vi "Dashboard Main.vi"() -> ()   [LabVIEW 2018]
uses:
  <vilib>/Rock Robotics/WPI/Camera/WPI_CameraSettings Read MJPG.ctl
  <vilib>/Rock Robotics/WPI/Camera/WPI_CameraImageSize.ctl
  <vilib>/Rock Robotics/WPI/Camera/WPI_CameraExposure Values.ctl
  <vilib>/Rock Robotics/WPI/Camera/WPI_CameraWhite Balance Values.ctl
  <vilib>/Utility/miscctls.llb/LVRowAndColumnTypeDef.ctl
  <vilib>/event_ctls.llb/eventvkey.ctl
  <vilib>/Rock Robotics/Network Tables/NT Read Numeric Array.vi
  <vilib>/Rock Robotics/WPI/Dashboard/WPI_DashboardLogging Global.vi
  <vilib>/Rock Robotics/Network Tables/NT Write Boolean.vi
  Vision Things/Dashboard globals.vi
  <vilib>/Utility/inputDevices.llb/keyboardAcquire.vi
  <vilib>/Rock Robotics/Network Tables/NT Write Variant.vi
panel:
  out "Time Remaining":sgl
  in  "Camera Settings Right":T1={"Frame Rate"=30, "Compression"=30, "Size"=1, "DB Camera Config"=FALSE} {"Frame Rate" scale=1.0..30.0; "Compression" scale=100.0..-1.0; "Size" items=["640x480", "320x240", "160x120"]}
  in  "Camera Name Right":string(combo)="No Camera Selection"
  out "Camera Perf":string
  in  "Camera Settings":T1={"Frame Rate"=30, "Compression"=30, "Size"=1, "DB Camera Config"=FALSE} {"Frame Rate" scale=1.0..30.0; "Compression" scale=100.0..-1.0; "Size" items=["640x480", "320x240", "160x120"]}
  in  "TCP":refnum<k5>
  in  "Rec Mode":enum32{"Stop", "Record", "Playback"}(radio)
  out "Robot IP":string
  out "Image Message":string="Timeout in Camera Communications"
  in  "Dashboard Tab":T2(tab)
  in  "Don't do Auton":bool
  in  "Desired Target":T3(radio)
  in  "Select Auto":string(combo)="Select Autonomous ..."
  out "NT Connection":bool
  out "MotorChart R":cluster{"Numeric":dbl, "Numeric":dbl}(graph)
  out "MotorChart L":cluster{"Numeric":dbl, "Numeric":dbl}(graph)
  out "MotorSliders R":cluster{"MotorSlide1":dbl, "MotorSlide2":dbl} {"MotorSlide2" scale=-1.0..1.0 scale format="%#_2e"; "MotorSlide1" scale=-1.0..1.0 scale format="%#_2e"}
  out "MotorSliders L":cluster{"MotorSlide1":dbl, "MotorSlide2":dbl} {"MotorSlide2" scale=-1.0..1.0 scale format="%#_2e"; "MotorSlide1" scale=-1.0..1.0 scale format="%#_2e"}
  out "Gyro":dbl(knob) scale=0.0..360.0
  out "JS1 Z":dbl(slide) scale=-1.0..1.0 scale format="%#_2e"
  out "JS1 Graph":cluster{"X":dbl, "Y":dbl}[](graph)
  out "JS1 Buttons":T4
  out "JS2 Z":dbl(slide) scale=-1.0..1.0 scale format="%#_2e"
  out "JS2 Graph":cluster{"X":dbl, "Y":dbl}[](graph)
  out "JS2 Buttons":T4
  out "Mode":T5(ring)=enum."Auto Disabled"
  out "Right Camera Perf":cluster{"Bandwidth (Mbps)":dbl, "FPS":dbl}
  in  "Auton Side":enum16{"Front", "Left", "Right"}(ring)
  in  "Side Code":enum16{"Right", "Left"}(ring)
  in  "Slot #":enum16{"3", "2", "1"}(ring)
  out "Auton String":string
  in  "Starting Postion":enum16{"2R", "2L", "1L", "1R", "1M"}(ring)
  in  "Camera 0 Settings":T6={"fps"=30, "compression"=30, "Image Size"=enum."320x240", "Config Shown"=FALSE}
  in  "Camera 1 Settings":T6={"fps"=30, "compression"=30, "Image Size"=enum."320x240", "Config Shown"=FALSE}
  out "Camera Image Right":T8(plugin-control)
  in  "DB/String 9":string
  in  "DB/String 8":string
  in  "DB/String 7":string
  in  "DB/String 6":string
  in  "DB/String 5":string
  in  "DB/String 4":string
  in  "DB/String 3":string
  in  "DB/String 2":string
  in  "DB/String 1":string
  in  "DB/String 0":string
  in  "DB/Slider 0":dbl(slide) scale=0.0..5.0
  in  "DB/Slider 1":dbl(slide) scale=0.0..5.0
  in  "DB/Slider 2":dbl(slide) scale=0.0..5.0
  in  "DB/Slider 3":dbl(slide) scale=0.0..5.0
  out "DB/LED 3":bool
  out "DB/LED 2":bool
  out "DB/LED 1":bool
  out "DB/LED 0":bool
  in  "DB/Button 3":bool
  in  "DB/Button 2":bool
  in  "DB/Button 1":bool
  in  "DB/Button 0":bool caption="New Name"
  in  "Test Slider":dbl(slide) scale=0.0..100.0 scale format="%#_3g"
  in  "On/Off":bool caption="Solenoid"
  in  "Test Name":u16(ring) items=["Select the test to run..."]
  in  "Test Tree":string(tree)
  in  "Motor":cluster{"Value":dbl, "Enable":bool} {"Value" scale=-1.0..1.0 scale format="%#_3g"}
  out "Progress":T9 {"Test Progress" scale=0.0..100.0}
  in  "Rev/Fwd":cluster{"Forward":bool, "Reverse":bool}
  in  "Test Ring":u16(ring) items=["Monochrome", "Color"]
  out "Cmd Status":string
  in  "Execute Command":bool
  in  "Command Params":string[][](table)
  in  "Command Selection":i32(listbox)
  in  "CheckList":i32(listbox)
  out "Tree":string(tree)
  out "Camera Image":T8(plugin-control)
  out "Background":bool
  in  "Camera Name":string(combo)="No Camera Selection"
  # "HW"
  # "HW"
  # "Joysticks"
  # "Drive Motors"
  # "Front"
  # "Right"
  # "Left"
  # "Back"
  # "This Tab intentionally left empty"
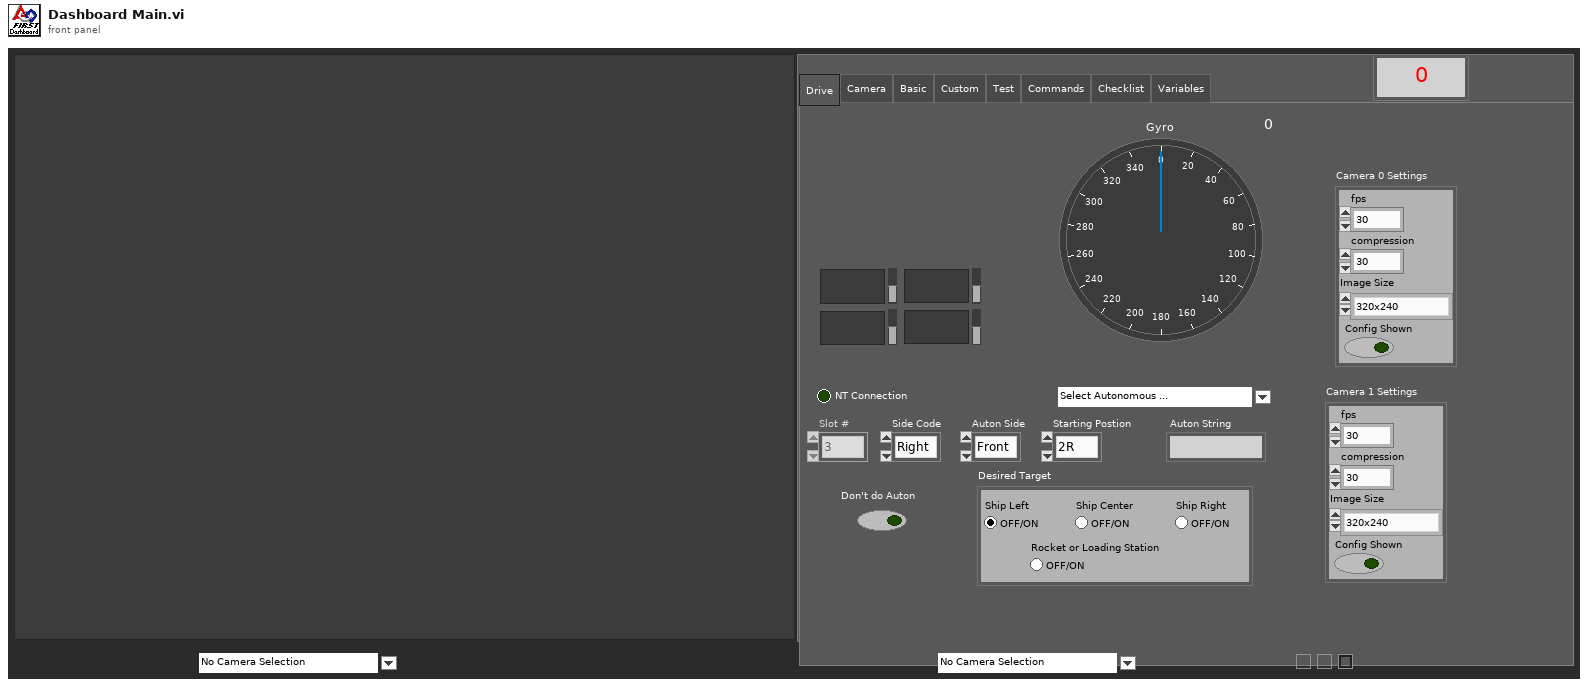
[diagram p1: front panel]
types:
  T1 = cluster{"Frame Rate":i32, "Compression":i32, "Size":u16, "DB Camera Config":bool}
  T2 = enum32{"Drive", "Camera", "Basic", "Custom", "Test", "Commands", "Checklist", "Variables"}
  T3 = enum32{"Ship Left", "Ship Center", "Ship Right", "Rocket or Loading Station"}
  T4 = cluster{bool, bool, bool, bool, bool, bool, bool, bool, bool, bool, bool, bool}
  T5 = enum8{"Tele-Op Disabled", "Tele-Op Enabled", "Auto Disabled", "Auto Enabled", "Test Disabled", "Test Enabled", "Disconnected", "No Code", "E-Stop"}
  T6 = typedef "WPI_CameraSettings Read MJPG.ctl" = cluster{"fps":i32, "compression":i32, "Image Size":T7, "Config Shown":bool}
  T7 = typedef "WPI_CameraImageSize.ctl" = enum16{"640x480", "320x240", "160x120", "Custom"}
  T8 = typedef "IMAQ Image.ctl" = refnum<image>
  T9 = cluster{"Test Progress":u8, "Test Progress Text":string}
  T10 = cluster{"Save Path":path, "Interval (s)":dbl, "Keep":i32}
  T11 = typedef "Image Type" = u32
  T12 = cluster{"IDs":cluster{"RPC field ID":u16, "Unique ID":u16}, "String":string}
  T13 = enum8{"Enabled", "Disabled", "Disabled and Grayed Out"}
  T14 = enum16{"0", "1", "2", "3", "4", "5", "6", "7", "8", "9", "A", "B", "C", "D", "E", "F", "G", "H", "I", "J", "K", "L", "M", "N", "O", "P", "Q", "R", "S", "T", "U", "V", "W", "X", "Y", "Z", "F1", "F2", "F3", "F4", "F5", "F6", "F7", "F8", "F9", "F10", "F11", "F12", "F13", "F14", "F15", "ADD", "BACK", "BACKSLASH", "CAPITAL", "COMMA", "DECIMAL", "DELETE", "DIVIDE", "DOWN", "END", "EQUALS", "ESCAPE", "GRAVE (`)", "HOME", "INSERT", "LBRACKET", "LCONTROL", "LEFT", "L ALT", "LSHIFT", "LWIN", "MINUS", "MULTIPLY", "NEXT", "NUMLOCK", "NUMPAD_0", "NUMPAD_1", "NUMPAD_2", "NUMPAD_3", "NUMPAD_4", "NUMPAD_5", "NUMPAD_6", "NUMPAD_7", "NUMPAD_8", "NUMPAD_9", "PAUSE", "PERIOD", "PRIOR (PG UP)", "RBRACKET", "RCONTROL", "RETURN", "RIGHT", "R ALT", "RSHIFT", "RWIN", "SCROLL", "SEMICOLON", "SLASH", "SPACE", "SUBTRACT", "TAB", "UP", "ENTER (num pad)", "' (quote)"}[]
  T15 = enum16{"0", "1", "2", "3", "4", "5", "6", "7", "8", "9", "A", "B", "C", "D", "E", "F", "G", "H", "I", "J", "K", "L", "M", "N", "O", "P", "Q", "R", "S", "T", "U", "V", "W", "X", "Y", "Z", "F1", "F2", "F3", "F4", "F5", "F6", "F7", "F8", "F9", "F10", "F11", "F12", "F13", "F14", "F15", "ADD", "BACK", "BACKSLASH", "CAPITAL", "COMMA", "DECIMAL", "DELETE", "DIVIDE", "DOWN", "END", "EQUALS", "ESCAPE", "GRAVE (`)", "HOME", "INSERT", "LBRACKET", "LCONTROL", "LEFT", "L ALT", "LSHIFT", "LWIN", "MINUS", "MULTIPLY", "NEXT", "NUMLOCK", "NUMPAD_0", "NUMPAD_1", "NUMPAD_2", "NUMPAD_3", "NUMPAD_4", "NUMPAD_5", "NUMPAD_6", "NUMPAD_7", "NUMPAD_8", "NUMPAD_9", "PAUSE", "PERIOD", "PRIOR (PG UP)", "RBRACKET", "RCONTROL", "RETURN", "RIGHT", "R ALT", "RSHIFT", "RWIN", "SCROLL", "SEMICOLON", "SLASH", "SPACE", "SUBTRACT", "TAB", "UP", "ENTER (num pad)", "' (quote)"}
  T16 = typedef "WPI_CameraExposure Values.ctl" = enum16{"Auto", "Flicker-free 50 Hz", "Flicker-free 60 Hz", "Hold current", "Custom"}
  T17 = typedef "WPI_CameraWhite Balance Values.ctl" = enum16{"Auto", "Fixed indoor", "Fixed outdoor 1", "Fixed outdoor 2", "Fixed fluorescent 1", "Fixed fluorescent 2", "Hold current", "Custom"}
  T18 = cluster{"Exposure":T16, "Exposure (%)":dbl, "Brightness":i32, "White Balance":T17, "Color Temp (K)":dbl}
  T19 = cluster{"Global Rectangle":i32[], "Contours":cluster{"Contour Type":u32, "ROI Type":u32, "Points":i32[]}[]}
  T20 = cluster{"Camera Name":string, string, "Saved DB Images Info":cluster{"Save Path":path, "Interval (s)":dbl, "Keep":i32}}
  T21 = cluster{"Camera Name Right":string, string, "Saved DB Images Info":cluster{"Save Path":path, "Interval (s)":dbl, "Keep":i32}}
  T22 = cluster{"Camera Image":refnum<vi>, "Dashboard Tab":refnum<vi>, "Background":refnum<vi>, "Rec Mode":refnum<vi>, "Test Slider":refnum<vi>, "On/Off ":refnum<vi>, "Test Ring":refnum<vi>, "Rev/Fwd":refnum<vi>, "Test Name":refnum<vi>, "Motor":refnum<vi>, "Progress":refnum<vi>, "CheckList":refnum<vi>, "Tree":refnum<vi>, "Test Tree":refnum<vi>, "Command Params":refnum<vi>, "Command Selection":refnum<vi>, "Execute Command":refnum<vi>, "Cmd Status":refnum<vi>, "Camera Settings":refnum<vi>, "Camera Name":refnum<vi>, "Camera Perf":refnum<vi>, "Camera Settings Right":refnum<vi>, "Camera Name Right":refnum<vi>, "Camera Image Right":refnum<vi>}
  T23 = cluster{"Error Strings":string, "Disable Counts":cluster{u16, u16}, "Rail Faults":cluster{u16, u16, u16}, "Robot IP":string, "DB Mode":u8, "Event Info":cluster{"Name":string, "Type":u8, "Number":u16, "Replay":u8}}
  T24 = cluster{"Storage":cluster{"Disk Free":u64, "RAM Block":u32, "RAM free":u32}, "CPU Utilization":cluster{"CPU % ISR":sgl, "CPU % Time Crit":sgl, "CPU % Timed Str":sgl, "CPU % High":sgl, "CPU % Above":sgl, "CPU % Normal":sgl, "CPU % Low":sgl}, "CAN":cluster{"% Bus Utilization":sgl, "Bus Off Cnt":u32, "TX_FIFO Full Cnt":u32, "Receive Error Cnt":u8, "Transmit Error Cnt":u8}, "HID":cluster{"HID Outputs":u32, "Rumble Low":u16, "Rumble High":u16}[]}
  T25 = cluster{"Status bits":cluster{"Test Mode":bool, "Autonomous":bool, "Enabled":bool, "Code Start":bool, "Brownout":bool, "Reserved 2":bool, "Reserved 3":bool, "E-Stop":bool}, "Code Trace":cluster{"Disabled":bool, "TeleOp":bool, "Auto":bool, "Test":bool}, "Controller Type":enum16{"unknown", "cRIO", "roboRio"}, "Code?":enum16{"unknown", "noCode", "code"}, "Battery V":dbl}
  T26 = cluster{"Control Bits":cluster{"TestMode":bool, "Autonomous":bool, "Enabled":bool, "FMS Present":bool, bool, bool, bool, "E-Stop":bool}, "Team Station ":u8, "Countdown":sgl, "Joystick Values":cluster{"Axes":dbl[], "Buttons":bool[], "POVs":i16[]}[]}
  T27 = cluster{"Increase in Left":dbl, "Increase in Right":dbl}[]
  T28 = cluster{"Axes":dbl[], "Buttons":bool[], "POVs":i16[]}[]
  T29 = cluster{"Axes":dbl[], "Buttons":bool[], "POVs":i16[]}
  T30 = cluster{"Buttons[0]":bool, "Buttons[1]":bool, "Buttons[2]":bool, "Buttons[3]":bool, "Buttons[4]":bool, "Buttons[5]":bool, "Buttons[6]":bool, "Buttons[7]":bool, "Buttons[8]":bool, "Buttons[9]":bool, "Buttons[10]":bool, "Buttons[11]":bool}
  T31 = cluster{"Operation":enum16{"Update", "Clear"}, "Color Box":u32}[]
  T32 = typedef "eventvkey.ctl" = enum16{"ASCII", "Enter", "Return", "Shift", "Ctrl", "Alt", "Cmd", "Opt", "Caps", "NumLock", "Clear", "Break", "Up", "Down", "Left", "Right", "Insert", "Delete", "Home", "End", "PageUp", "PageDown", "Escape", "Help", "Pause", "ScrollLock", "F1", "F2", "F3", "F4", "F5", "F6", "F7", "F8", "F9", "F10", "F11", "F12", "F13", "F14", "F15", "F16", "F17", "F18", "F19", "F20", "F21", "F22", "F23", "F24", "Play", "VolumeUp", "VolumeDown", "Mute", "Two Byte Char"}
  T33 = cluster{"Image Size":bool, "Image Type":bool, "Pixel Value":bool, "ROI Information":bool, "Zoom Factor":bool}
  T34 = cluster{"Operation":enum16{"Update", "Clear"}, "Color Box":u32}
  T35 = typedef "LVRowAndColumnTypeDef.ctl" = cluster{"Row":i32, "Column":i32}
  T36 = cluster{"Shift":bool, "Ctrl":bool, "Alt":bool, "Cmd":bool, "Opt":bool}
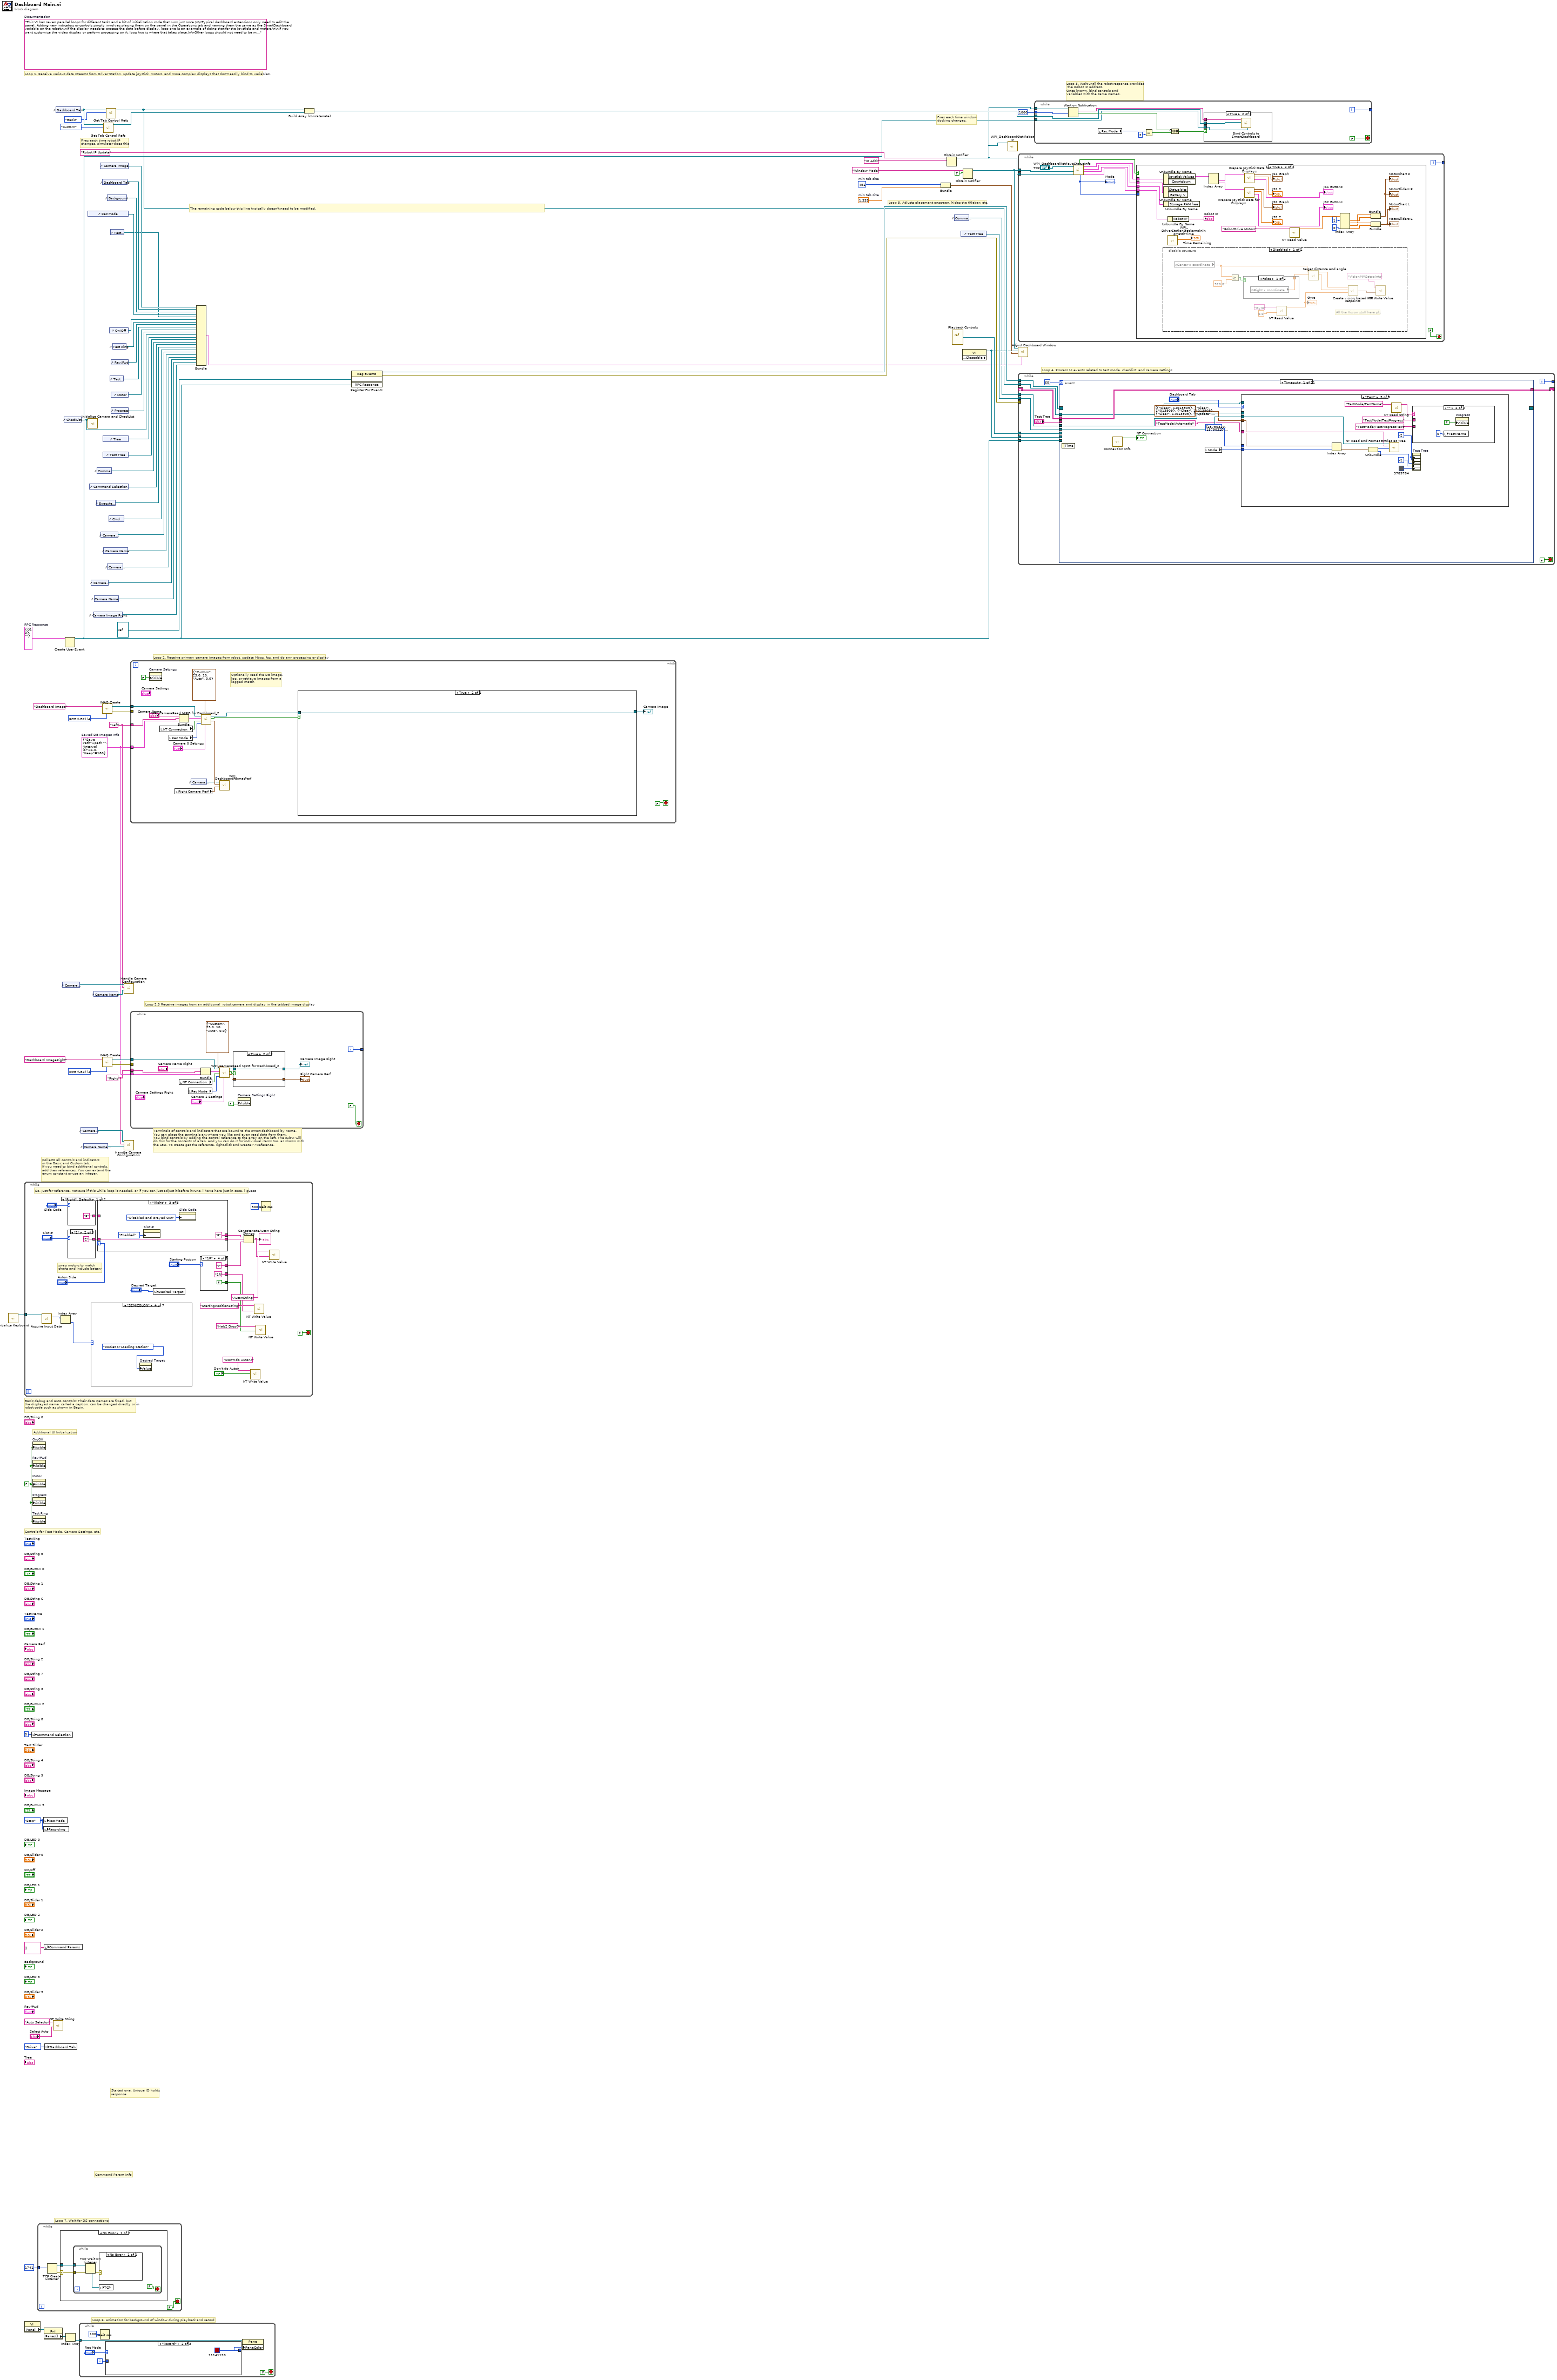
[diagram p0: block diagram]
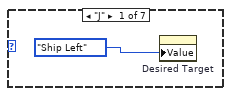
[diagram p2: hidden frame]
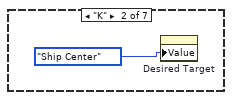
[diagram p3: hidden frame]
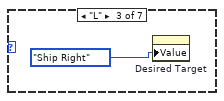
[diagram p4: hidden frame]
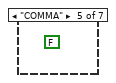
[diagram p5: hidden frame]
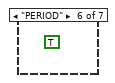
[diagram p6: hidden frame]
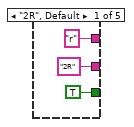
[diagram p8: hidden frame]
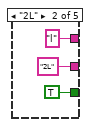
[diagram p9: hidden frame]
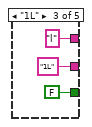
[diagram p10: hidden frame]
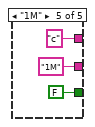
[diagram p11: hidden frame]
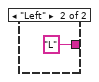
[diagram p12: hidden frame]
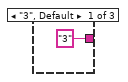
[diagram p13: hidden frame]
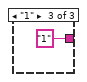
[diagram p14: hidden frame]
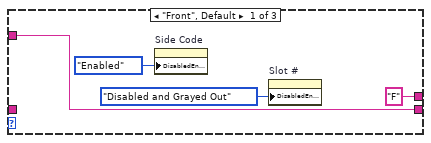
[diagram p15: hidden frame]
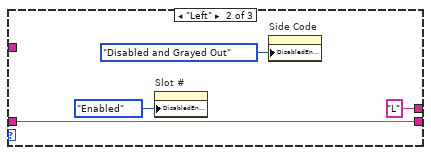
[diagram p16: hidden frame]
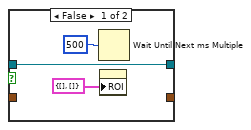
[diagram p17: hidden frame]
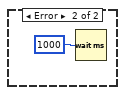
[diagram p18: hidden frame]
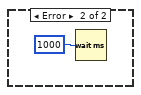
[diagram p19: hidden frame]
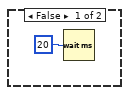
[diagram p20: hidden frame]
diagram:
  w5 = T10 {"Save Path"=path "", "Interval (s)"=1.0, "Keep"=180}  # Saved DB Images Info
  w4 = "Right"
  w3 = "Left"
  w15 = T11 4 items=["Grayscale (U8)", "Grayscale (I16)", "Grayscale (SGL)", "Complex (CSG)", "RGB (U32)", "HSL (U32)", "RGB (U64)"] ("Image Type")
  w31 = T12 {"IDs"={"RPC field ID"=0, "Unique ID"=0}, "String"=""}  # RPC Response
  w53 = 491  # min tab size
  w52 = 1.333  # min tab size
  w60 = enum32{"Stop", "Record", "Playback"}."Stop" ("Rec Mode")
  w37 = FALSE ("Visible")
  (unwired) "This VI has seven parallel loops for different tasks and a bit of initialization code that runs just once.\n\nTypical dashboard extensions only need to edit the panel. Adding new indicators or controls simply involves placing them on the panel in the Operations tab and naming them the same as the SmartDashboard variable on the robot\n\nIf the display needs to process the data before display, loop one is an example of doing that for the joysticks and motors.\n\nIf you want customize the video display or perform processing on it, loop two is where that takes place.\n\nOther loops should not need to be modified. They are pretty standard, and document the task they perform."  # Documentation
  w77 = T11 4 items=["Grayscale (U8)", "Grayscale (I16)", "Grayscale (SGL)", "Complex (CSG)", "RGB (U32)", "HSL (U32)", "RGB (U64)"] ("Image Type")
  # "Collects all controls and indicators\nin the Basic and Custom tab.\nIf you need to bind additional controls,\nadd their references. You can extend the\nenum constant or use an integer."
  # "Terminals of controls and indicators that are bound to the smart dashboard by name.\nYou can place the terminals anywhere you like and even read data from them.\nYou bind controls by adding the control reference to the array on the left. The subVI will\ndo this for the contents of a tab, and you can do it for individual items too, as shown with\nthe LED. To create get the reference, right-click and Create>>Reference."
  # "Loop 2.5 Receive images from an additional  robot camera and display in the tabbed image display"
  # "Command Param Info"
  # "Started one, Unique ID holds\nresponse"
  # "Loop 7. Wait for DS connections"
  # "Basic debug and auto controls: Their data names are fixed, but\nthe displayed name, called a caption, can be changed directly or in\nrobot code such as shown in Begin."
  # "Controls for Test Mode, Camera Settings, etc."
  # "Additional UI Initialization"
  # "Loop 6. Animation for background of window during playback and record"
  # "Fires each time robot IP\nchanges, simulator does this"
  # "Fires each time window\ndocking changes."
  # "The remaining code below this line typically doesn't need to be modified."
  # "Loop 4. Process UI events related to test mode, checklist, and camera settings"
  # "Loop 3. Wait until the robot response provides\n the Robot IP address.\nOnce known, bind controls and\nvariables with the same names."
  # "Loop 5. Adjusts placement onscreen, hides the titlebar, etc."
  # "Loop 1. Receive various data streams from Driver Station, update joystick, motors, and more complex displays that don't easily bind to variables."
  # "Loop 2. Receive primary camera images from robot, update Mbps, fps, and do any processing or display"
  n1 = call <vilib>:"Intialize Keyboard.vi"() -> ("device ID"=w2:refnum<k1>)  [unwired: 10 in, 1 out]
  n2 = while {
    tunnel: w2 -> [w84]
    stop <- FALSE stop-if-true
    # "So, Just for reference, not sure if this while loop is needed, or if you can just adjust it before it runs, i have here just in case, i guess"
    # "swap motors to match\ncharts and include battery"
    n3 = call-poly <vilib>:"Acquire Input Data.vi"("device ID"=w84) -> ("keys pressed"=w83:T14)  [unwired: 16 in, 2 out]
    n4 = Index Array(array=w83) -> (element=w82:T15)  [unwired: 1 in]
    n5 = case shown="\"Right\", Default" "Side Code" {
      tunnel: ["R" "L"] -> w96
      frame "Right", Default {
      }
      frame "Left" {
      }
    }
    n6 = case shown="\"2\"" "Slot #" {
      tunnel: ["3" "2" "1"] -> w97
      frame "3", Default {
      }
      frame "2" {
      }
      frame "1" {
      }
    }
    n7 = case shown="\"SEMICOLON\"" w82 {
      frame "J" {
        n8 = property on="Desired Target" class="RadioBtnsControl (strict)"("Value"=T3."Ship Left" ("Desired Target")) -> ()  [unwired: 2 in, 2 out]
      }
      frame "K" {
        n9 = property on="Desired Target" class="RadioBtnsControl (strict)"("Value"=T3."Ship Center" ("Desired Target")) -> ()  [unwired: 2 in, 2 out]
      }
      frame "L" {
        n10 = property on="Desired Target" class="RadioBtnsControl (strict)"("Value"=T3."Ship Right" ("Desired Target")) -> ()  [unwired: 2 in, 2 out]
      }
      frame "SEMICOLON" {
        n11 = property on="Desired Target" class="RadioBtnsControl (strict)"("Value"=T3."Rocket or Loading Station" ("Desired Target")) -> ()  [unwired: 2 in, 2 out]
      }
      frame "COMMA" {
        (unwired) FALSE ("Enable Vision Processing")
      }
      frame "PERIOD" {
        (unwired) TRUE ("Enable Vision Processing")
      }
      frame "0", Default {
      }
    }
    n12 = case shown="\"Right\"" "Auton Side" {
      tunnel: w97 -> [_ w129 w133]
      tunnel: w96 -> [w125 _ _]
      tunnel: [w125 w129 w133] -> w92
      tunnel: ["F" "L" "R"] -> w93
      frame "Front", Default {
        n13 = property on="Side Code" class="Enum (strict)"("DisabledEnum"=T13."Enabled" ("Disabled")) -> ()  [unwired: 2 in, 2 out]
        n14 = property on="Slot #" class="Enum (strict)"("DisabledEnum"=T13."Disabled and Grayed Out" ("Disabled")) -> ()  [unwired: 2 in, 2 out]
      }
      frame "Left" {
        n15 = property on="Slot #" class="Enum (strict)"("DisabledEnum"=T13."Enabled" ("Disabled")) -> ()  [unwired: 2 in, 2 out]
        n16 = property on="Side Code" class="Enum (strict)"("DisabledEnum"=T13."Disabled and Grayed Out" ("Disabled")) -> ()  [unwired: 2 in, 2 out]
      }
      frame "Right" {
        n17 = property on="Slot #" class="Enum (strict)"("DisabledEnum"=T13."Enabled" ("Disabled")) -> ()  [unwired: 2 in, 2 out]
        n18 = property on="Side Code" class="Enum (strict)"("DisabledEnum"=T13."Disabled and Grayed Out" ("Disabled")) -> ()  [unwired: 2 in, 2 out]
      }
    }
    n19 = global write "Dashboard globals.vi" "Desired Target"("Desired Target") -> ()
    n20 = case shown="\"1R\"" "Starting Postion" {
      tunnel: ["2R" "2L" "1L" "1R" "1M"] -> w89
      tunnel: [TRUE TRUE FALSE FALSE FALSE] -> w86
      tunnel: ["r" "l" "l" "r" "c"] -> w85
      frame "2R", Default {
      }
      frame "2L" {
      }
      frame "1L" {
      }
      frame "1R" {
      }
      frame "1M" {
      }
    }
    n21 = Concatenate Strings(w93, w92, w85) -> (w90:string)
    "Auton String" <- w90
    n22 = call-poly <vilib>:"NT Write Value.vi"("Boolean"="Don't do Auton", "Name"="Don't do Auton?") -> ()  [unwired: 9 in, 1 out]
    n23 = call-poly <vilib>:"NT Write Value.vi"("String"=w89, "Name"="StartingPositionString") -> ()  [unwired: 9 in, 1 out]
    n24 = call-poly <vilib>:"NT Write Value.vi"("Boolean"=w86, "Name"="Hab2 Drop?") -> ()  [unwired: 9 in, 1 out]
    n25 = Wait (ms)(milliseconds to wait=u32 500) -> ()  [unwired: 1 out]
    n26 = call-poly <vilib>:"NT Write Value.vi"("String"=w90, "Name"="AutonString") -> ()  [unwired: 9 in, 1 out]
  }
  n27 = property class="VI"() -> ("Panel"=w67:refnum<vi>)  [unwired: 2 in, 2 out]
  n28 = local write "Command Selection"(u16 0 ("milliseconds to wait")) -> ()
  n29 = property on="On/Off" class="Bool (strict)"("Visible"=w37) -> ()  [unwired: 2 in, 2 out]
  n30 = property on="Rev/Fwd" class="Clust (strict)"("Visible"=w37) -> ()  [unwired: 2 in, 2 out]
  n31 = property on="Motor" class="Clust (strict)"("Visible"=w37) -> ()  [unwired: 2 in, 2 out]
  n32 = property on="Progress" class="Clust (strict)"("Visible"=w37) -> ()  [unwired: 2 in, 2 out]
  n33 = property on="Test Ring" class="Ring (strict)"("Visible"=w37) -> ()  [unwired: 2 in, 2 out]
  n34 = while {
    tunnel: u16 1741 ("timeout ms (25000)") -> [w138]
    stop <- FALSE stop-if-true
    n35 = TCP Create Listener(10:w138) -> (0:w137:errorcluster, 3:w139:refnum<k5>)  [unwired: 4 in, 1 out]
    n36 = case shown="No Error" w137 {
      selector: w137 -> [w141 _]
      tunnel: w139 -> [w142 _]
      frame No Error {
        n37 = while {
          tunnel: w142 -> [w145]
          tunnel: w141 -> [w144]
          stop <- FALSE stop-if-true
          n38 = TCP Wait On Listener(8:w144, 11:w145) -> (0:w146:errorcluster, 4:w147:refnum<k5>)  [unwired: 2 in, 3 out]
          n39 = case shown="No Error" w146 {
            frame No Error {
            }
            frame Error {
              n40 = Wait (ms)(milliseconds to wait=u32 1000) -> ()  [unwired: 1 out]
            }
          }
          n41 = local write "TCP"(w147) -> ()
        }
      }
      frame Error {
        n42 = Wait (ms)(milliseconds to wait=u32 1000) -> ()  [unwired: 1 out]
      }
    }
  }
  n43 = local write "Rec Mode"(w60) -> ()
  n44 = global write "WPI_DashboardLogging Global.vi" "Recording"(w60) -> ()
  n45 = property class="Pnl"(reference=w67) -> ("Panes[]"=w68:refnum<vi>[])  [unwired: 1 in, 2 out]
  n46 = local write "Command Params"(string[][] [] ("Command Params")) -> ()
  n47 = local write "Dashboard Tab"(T2."Drive" ("Dashboard Tab")) -> ()
  n48 = call <vilib>:"NT Write String.vi"("String"="Select Auto", "Name"="Auto Selector") -> ()  [unwired: 9 in, 1 out]
  n49 = control-ref of="Dashboard Tab"() -> (w58:refnum<vi>)
  n50 = control-ref of="Camera Settings"() -> (w24:refnum<vi>)
  n51 = control-ref of="CheckList"() -> (w48:refnum<vi>)
  n52 = Create User Event(user event datatype=w31) -> (user event=w27:refnum<user-event>)  [unwired: 1 in, 1 out]
  n53 = Index Array(array=w68) -> (element=w66:refnum<vi>)  [unwired: 1 in]
  n54 = while {
    tunnel: w66 -> [w151]
    i -> [w154]
    stop <- FALSE stop-if-true
    n55 = Wait (ms)(milliseconds to wait=u32 100) -> ()  [unwired: 1 out]
    n56 = case shown="\"Record\"" "Rec Mode" {
      tunnel: w154 -> [_ _ w169]
      tunnel: [u32 2829099 ("Base Color") u32 11141120 ("Target Color") w158] -> w150
      frame "Stop", Default {
        # "Reset the color, extra updates don't cost much"
      }
      frame "Record" {
      }
      frame "Playback" {
        # "Playback"
        n57 = Quotient & Remainder(x=w169, y=u32 50 ("milliseconds to wait")) -> (x-y*floor(x/y)=w165:u32)  [unwired: 1 out]
        n58 = Divide(x=w165, y=u32 50 ("milliseconds to wait")) -> (x/y=w162:dbl)
        n59 = Multiply(x=6.283185307179586, y=w162) -> (x*y=w167:dbl)
        n60 = Sine(x=w167) -> (sin(x)=w166:dbl)
        n61 = Absolute Value(x=w166) -> (abs(x)=w159:dbl)
        n62 = call "Interpolate RGB Color.vi"("Proportion"=w159, "Target Color"=u32 30976, "Base Color"=u32 2829099) -> ("Result Color"=w158:u32)  [unwired: 8 in]
      }
    }
    n63 = property class="Pane"(reference=w151, "PaneColor"=w150) -> ()  [unwired: 1 in, 2 out]
  }
  n64 = control-ref of="Camera Settings Right"() -> (w12:refnum<vi>)
  n65 = control-ref of="Camera Name Right"() -> (w11:refnum<vi>)
  n66 = control-ref of="Rec Mode"() -> (w43:refnum<vi>)
  n67 = call "Initialize Camera and CheckList.vi"("ListBox in"=w48) -> ()  [unwired: 11 in]
  n68 = control-ref of="Command Selection"() -> (w30:refnum<vi>)
  n69 = control-ref of="Camera Settings Right"() -> (w10:refnum<vi>)
  n70 = control-ref of="Camera Image Right"() -> (w8:refnum<vi>)
  n71 = control-ref of="Camera Name"() -> (w23:refnum<vi>)
  n72 = control-ref of="Camera Name Right"() -> (w9:refnum<vi>)
  n73 = control-ref of="Execute Command"() -> (w32:refnum<vi>)
  n74 = control-ref of="Command Params"() -> (w33:refnum<vi>)
  n75 = control-ref of="Camera Image"() -> (w55:refnum<vi>)
  n76 = control-ref of="Camera Settings"() -> (w22:refnum<vi>)
  n77 = control-ref of="Dashboard Tab"() -> (w54:refnum<vi>)
  n78 = call "IMAQ Create"("Image Name"="Dashboard Image", "Image Type"=w77) -> ("New Image"=w75:T8, "error out"=w74:errorcluster)  [unwired: 2 in, 1 out]
  n79 = call "IMAQ Create"("Image Name"="Dashboard ImageRight", "Image Type"=w15) -> ("New Image"=w14:T8, "error out"=w13:errorcluster)  [unwired: 2 in, 1 out]
  n80 = control-ref of="Tree"() -> (w47:refnum<vi>)
  n81 = control-ref of="Test Tree"() -> (w46:refnum<vi>)
  n82 = call <vilib>:"Get Tab Control Refs.vi"("Page Index"=T2."Custom" ("Dashboard Tab"), "TabControl in"=w58) -> ("ControlsOnPage"=w57:refnum<vi>[])  [unwired: 9 in]
  n83 = control-ref of="Camera Name"() -> (w21:refnum<vi>)
  n84 = call <vilib>:"Get Tab Control Refs.vi"("Page Index"=T2."Basic" ("Dashboard Tab"), "TabControl in"=w58) -> ("ControlsOnPage"=w19:refnum<vi>[])  [unwired: 9 in]
  n85 = control-ref of="Background"() -> (w50:refnum<vi>)
  n86 = control-ref of="Camera Perf"() -> (w20:refnum<vi>)
  n87 = control-ref of="Cmd Status"() -> (w26:refnum<vi>)
  n88 = control-ref of="On/Off"() -> (w41:refnum<vi>)
  n89 = control-ref of="Test Name"() -> (w45:refnum<vi>)
  n90 = control-ref of="Test Slider"() -> (w42:refnum<vi>)
  n91 = control-ref of="Rev/Fwd"() -> (w39:refnum<vi>)
  n92 = control-ref of="Motor"() -> (w44:refnum<vi>)
  n93 = control-ref of="Progress"() -> (w38:refnum<vi>)
  n94 = control-ref of="Test Ring"() -> (w40:refnum<vi>)
  n95 = call "Handle Camera Configuration.vi"("CameraNameRef"=w23, "Display Name"=w3, "ClusterRef"=w24) -> ()  [unwired: 9 in]
  n96 = call "Handle Camera Configuration.vi"("CameraNameRef"=w11, "Display Name"=w4, "ClusterRef"=w12) -> ()  [unwired: 9 in]
  n97 = while {
    tunnel: w75 -> [w185]
    tunnel: w74 -> [_]
    tunnel: w5 -> [w179]
    tunnel: w3 -> [w176]
    stop <- FALSE stop-if-true
    # "Optionally read the DB image,\nlog, or retrieve images from a\nlogged match"
    n98 = property on="Camera Settings" class="Clust (strict)"("Visible"=FALSE) -> ()  [unwired: 2 in, 2 out]
    n99 = local read "NT Connection"() -> (w180:bool)
    n100 = local read "Rec Mode"() -> (w182:enum32{"Stop", "Record", "Playback"})
    n101 = local read "Right Camera Perf"() -> (w174:cluster{"Bandwidth (Mbps)":dbl, "FPS":dbl})
    n102 = Bundle("Camera Name"="Camera Name", w176, "Saved DB Images Info"=w179) -> (w178:T20)  [unwired: 1 in]
    n103 = control-ref of="Camera Perf"() -> (w173:refnum<vi>)
    n104 = call <vilib>:"WPI_CameraRead MJPG for Dashboard_2.vi"("Camera Settings"="Camera 0 Settings", "Camera Settings 2"=T18 {"Exposure"=enum."Custom", "Exposure (%)"=25.0, "Brightness"=10, "White Balance"=enum."Auto", "Color Temp (K)"=0.0}, "Rec Mode"=w182, "NT Connection"=w180, "Capture Info"=w178, "Image in"=w185) -> ("perf info"=w175:cluster{"Bandwidth (Mbps)":dbl, "fps":dbl}, "Active"=w183:bool, "Image\\ out"=w184:T8)  [unwired: 3 in]
    n105 = call <vilib>:"WPI_DashboardFormatPerf.vi"("Right Camera Perf"=w174, "Performance"=w175, "String in"=w173) -> ()  [unwired: 9 in]
    n106 = case shown="True" w183 {
      tunnel: w184 -> [w188 w190]
      tunnel: [w188 w190] -> w181
      frame False {
        # "Sleep for 500ms"
        n107 = Wait Until Next ms Multiple(millisecond multiple=u32 500) -> ()  [unwired: 1 out]
        n108 = property on="Camera Image" class="ImageControl"("ROI"=T19 {"Global Rectangle"=[], "Contours"=[]}) -> ()  [unwired: 2 in, 2 out]
      }
      frame True {
      }
    }
    "Camera Image" <- w181
  }
  n109 = while {
    tunnel: w14 -> [w207]
    tunnel: w13 -> [_]
    tunnel: [w203] -> _
    tunnel: w5 -> [w199]
    tunnel: w4 -> [w196]
    i -> [w203]
    stop <- FALSE stop-if-true
    n110 = local read "NT Connection"() -> (w200:bool)
    n111 = local read "Rec Mode"() -> (w206:enum32{"Stop", "Record", "Playback"})
    n112 = Bundle("Camera Name Right"="Camera Name Right", w196, "Saved DB Images Info"=w199) -> (w198:T21)  [unwired: 1 in]
    n113 = call <vilib>:"WPI_CameraRead MJPG for Dashboard_2.vi"("Camera Settings"="Camera 1 Settings", "Camera Settings 2"=T18 {"Exposure"=enum."Custom", "Exposure (%)"=25.0, "Brightness"=10, "White Balance"=enum."Auto", "Color Temp (K)"=0.0}, "Rec Mode"=w206, "NT Connection"=w200, "Capture Info"=w198, "Image in"=w207) -> ("perf info"=w194:cluster{"Bandwidth (Mbps)":dbl, "fps":dbl}, "Active"=w202:bool, "Image\\ out"=w205:T8)  [unwired: 3 in]
    n114 = case shown="True" w202 {
      tunnel: w205 -> [w209 w212]
      tunnel: [w209 w212] -> w201
      tunnel: [_ w211] -> w195
      tunnel: w194 -> [_ w211]
      frame False {
        n115 = Wait Until Next ms Multiple(millisecond multiple=u32 500) -> ()  [unwired: 1 out]
        n116 = property on="Camera Image Right" class="ImageControl"("ROI"=T19 {"Global Rectangle"=[], "Contours"=[]}) -> ()  [unwired: 2 in, 2 out]
      }
      frame True {
      }
    }
    "Camera Image Right" <- w201
    "Right Camera Perf" <- w195
    n117 = property on="Camera Settings Right" class="Clust (strict)"("Visible"=FALSE) -> ()  [unwired: 2 in, 2 out]
  }
  n118 = Bundle("Camera Image"=w55, "Dashboard Tab"=w54, "Background"=w50, "Rec Mode"=w43, "Test Slider"=w42, "On/Off"=w41, "Test Ring"=w40, "Rev/Fwd"=w39, "Test Name"=w45, "Motor"=w44, "Progress"=w38, "CheckList"=w48, "Tree"=w47, "Test Tree"=w46, "Command Params"=w33, "Command Selection"=w30, "Execute Command"=w32, "Cmd Status"=w26, "Camera Settings"=w22, "Camera Name"=w21, "Camera Perf"=w20, "Camera Settings Right"=w10, "Camera Name Right"=w9, "Camera Image Right"=w8) -> (w49:T22)  [unwired: 1 in]
  n119 = Build Array (concatenate)(w19, w57) -> (w56:refnum<vi>[])
  n120 = register-events(refnum<vi> refnum, w27) -> (reference out=w64:refnum<event-registration>, error out=w63:errorcluster)  [unwired: 2 in]
  n121 = Bundle("min tab size"=w53, "min tab size"=w52) -> (w51:cluster{"min tab size":i32, "min tab size":dbl})  [unwired: 1 in]
  n122 = Obtain Notifier(name (unnamed)="Robot IP Update", notification data type="IP Addr" ("name (unnamed)")) -> (notifier out=w1:refnum<notifier>)  [unwired: 2 in, 2 out]
  n123 = vi-ref "Playback Controls.vi"() -> (w65:refnum<vi>)
  n124 = control-ref of="Command Params"() -> (w25:refnum<vi>)
  n125 = control-ref of="Test Tree"() -> (w69:refnum<vi>)
  n126 = property class="VI" props=["Front Panel.Closeable"]() -> (reference out=w59:refnum<vi>)  [unwired: 2 in, 2 out]
  n127 = Obtain Notifier(name (unnamed)="Window Mode", notification data type=TRUE) -> (notifier out=w36:refnum<notifier>)  [unwired: 2 in, 2 out]
  n128 = call "WPI_DashboardGet Robot IP.vi"("Notifier in"=w1) -> ()  [unwired: 11 in]
  n129 = while {
    tunnel: [w222] -> _
    tunnel: w1 -> [w216]
    tunnel: w36 -> [w213]
    i -> [w222]
    stop <- FALSE stop-if-true
    n130 = call <vilib>:"WPI_DashboardRetrieveStatusInfo.vi"("Binding Refnum"=w216, "Window Mode Notifier"=w213, "TCP Cnx"="TCP") -> ("Power and Errors"=w217:T23, "Robot Metrics"=w220:T24, "Status Info"=w221:T25, "Control Info"=w218:T26, "Robot Mode"=w215:T5, "Process?"=w219:bool)  [unwired: 3 in]
    "Mode" <- w215
    n131 = case shown="True" w219 {
      tunnel: w221 -> [_ w249]
      tunnel: w220 -> [_ w248]
      tunnel: w218 -> [_ w247]
      tunnel: w217 -> [_ w246]
      tunnel: w215 -> [_ _]
      frame False {
        n132 = Wait (ms)(milliseconds to wait=u32 20) -> ()  [unwired: 1 out]
      }
      frame True {
        n133 = disable-structure shown="Disabled" {
          frame Disabled {
            # "All the Vision stuff here plz"
            n134 = global read "Dashboard globals.vi" "Center x coordinate"() -> (w251:sgl)
            n135 = Greater Or Equal?(x=w251, y=sgl 320.0) -> (x >= y?=w253:bool)
            n136 = case shown="False" w253 {
              tunnel: [w261 w262] -> w250
              frame False {
                n137 = global read "Dashboard globals.vi" "Right x coordinate"() -> (w261:sgl)
              }
              frame True {
                n138 = global read "Dashboard globals.vi" "Left x coordinate"() -> (w262:sgl)
              }
            }
            n139 = call-poly <vilib>:"NT Read Value.vi"("Default Value"=0.0, "Name"="Gyro") -> ("Numeric"=w256:dbl)  [unwired: 8 in, 1 out]
            "Gyro" <- w256
            n140 = call "target distance and angle.vi"("x side"=w250, "x center"=w251) -> ("target angle in degrees"=w254:dbl, "distance from target in inches"=w255:dbl)  [unwired: 8 in]
            n141 = call "Create vision based MM setpoints.vi"("Gyro"=w256, "(phi) Vision's angle that the target is offcenter"=w254, "(I) Vision's distance to target"=w255) -> ("Vision-based MM Setpoints"=w259:T27)  [unwired: 1 in]
            n142 = call-poly <vilib>:"NT Write Value.vi"("Variant"=w259, "Name"="VisionMMSetpoints") -> ()  [unwired: 9 in, 1 out]
          }
          frame Enabled {
          }
        }
        n143 = Unbundle By Name(w247) -> ("Joystick Values"=w237:T28)  [unwired: 1 out]
        n144 = Unbundle By Name(w249) -> ()  [unwired: 2 out]
        n145 = Unbundle By Name(w248) -> ()  [unwired: 1 out]
        n146 = Unbundle By Name(w246) -> ("Robot IP"=→"Robot IP":string)
        n147 = call <vilib>:"WPI_DriverStationGetRemainingMatchTime.vi"() -> ("Match Time(s)"=→"Time Remaining":sgl)  [unwired: 10 in, 1 out]
        n148 = Index Array(array=w237) -> (element #1=w236:T29, element #2=w232:T29)  [unwired: 2 in]
        n149 = call "Prepare Joystick Data for Displays.vi"("Joystick Values"=w236) -> ("Buttons"=→"JS1 Buttons":T30, "Z Axis"=→"JS1 Z":dbl, "Cartesian Data"=→"JS1 Graph":cluster{"X axis":dbl, "X axis":dbl}[])  [unwired: 8 in]
        n150 = call "Prepare Joystick Data for Displays.vi"("Joystick Values"=w232) -> ("Buttons"=→"JS2 Buttons":T30, "Z Axis"=→"JS2 Z":dbl, "Cartesian Data"=→"JS2 Graph":cluster{"X axis":dbl, "X axis":dbl}[])  [unwired: 8 in]
        n151 = call-poly <vilib>:"NT Read Value.vi"("Name"="RobotDrive Motors") -> ("Numeric Array"=w227:dbl[])  [unwired: 9 in, 1 out]
        n152 = Index Array(array=w227, index #1=1, index #4=0) -> (element #1=w241:dbl, element #2=w242:dbl, element #3=w240:dbl, element #4=w245:dbl)  [unwired: 2 in]
        n153 = Bundle("Numeric"=w240, "Numeric"=w241) -> (→"MotorChart R" →"MotorSliders R":cluster{"Numeric":dbl, "Numeric":dbl})  [unwired: 1 in]
        n154 = Bundle("Numeric"=w242, "Numeric"=w245) -> (→"MotorChart L" →"MotorSliders L":cluster{"Numeric":dbl, "Numeric":dbl})  [unwired: 1 in]
      }
    }
  }
  n155 = call "Adjust Dashboard Window.vi"("Sizing Refnums"=w49, "Size Constraints"=w51, "VI"=w59, "WIn Mode"=w36) -> ()  [unwired: 8 in]
  n156 = while {
    tunnel: [w272] -> _
    tunnel: w69 -> [w271]
    tunnel: w65 -> [w270]
    tunnel: w64 -> [w269]
    tunnel: w63 -> [_]
    tunnel: w59 -> [w268]
    tunnel: w27 -> [w267]
    tunnel: w25 -> [w266]
    shift-right: [w265] -> _
    shift-left: _ -> [w264]
    tunnel: w19 -> [w263]
    i -> [w272]
    stop <- FALSE stop-if-true
    n157 = event shown="[0] Timeout" {
      selector: w269 -> [_ _ _ _ _ _ _ _ _ _ _ _ _ _ _ _ _ _ _ _ _]
      dyn-events: [_ _ _ _ _ _ _ _ _ _ _ _ _ _ _ _ w532 _ _ _ _] -> _
      timeout: u32 60 ("milliseconds to wait") -> [_ _ _ _ _ _ _ _ _ _ _ _ _ _ _ _ _ _ _ _ _]
      tunnel: w271 -> [w284 _ _ _ _ _ _ _ _ _ _ _ _ _ _ _ _ _ _ _ _]
      tunnel: "Test Tree" -> [_ _ _ _ _ _ _ _ _ _ _ w499 w507 w509 w513 w521 _ _ _ _ _]
      tunnel: w270 -> [_ _ _ _ _ _ _ _ _ _ _ _ _ _ _ _ w534 _ w552 _ _]
      tunnel: w268 -> [_ _ _ _ _ _ _ _ _ _ _ _ _ _ _ _ w530 _ _ _ _]
      tunnel: w267 -> [_ _ _ _ _ _ _ _ _ _ _ _ _ _ _ _ w528 _ _ _ _]
      tunnel: w266 -> [w279 _ _ _ _ _ w450 _ _ _ _ _ _ _ _ _ _ _ _ _ _]
      tunnel: [w278 w327 w429 w434 w443 w447 w448 w457 w467 w474 w486 w498 w505 w508 w512 w520 w527 w547 w549 w553 w566] -> w265
      tunnel: w264 -> [w278 w327 w429 w434 w443 w447 w448 _ _ w474 w486 w498 w505 w508 w512 w520 w527 w547 w549 w553 w566]
      tunnel: w263 -> [w276 _ _ _ _ _ _ _ _ _ _ _ _ _ _ _ _ _ _ _ _]
      event Timeout {
        n158 = event-data() -> ()  [unwired: 1 in, 1 out]
        n159 = call <vilib>:"Connextion Info.vi"() -> ("Connected"=→"NT Connection":bool)  [unwired: 10 in, 1 out]
        n160 = local read "Mode"() -> (w281:T5)
        n161 = case shown="\"Test\"" "Dashboard Tab" {
          tunnel: w284 -> [_ _ w300 _ _]
          tunnel: "TestMode/Automatic/" ("Name Pattern") -> [_ _ w299 _ _]
          tunnel: T31 [{"Operation"=enum."Clear", "Color Box"=14013909}, {"Operation"=enum."Clear", "Color Box"=14013909}, {"Operation"=enum."Clear", "Color Box"=14013909}, {"Operation"=enum."Clear", "Color Box"=14013909}, {"Operation"=enum."Update", "Color Box"=14013909}, {"Operation"=enum."Update", "Color Box"=16777215}, {"Operation"=enum."Clear", "Color Box"=14013909}, {"Operation"=enum."Clear", "Color Box"=14013909}, {"Operation"=enum."Clear", "Color Box"=14013909}] -> [_ _ w292 _ w320]
          tunnel: w281 -> [_ _ w291 _ w319]
          tunnel: u32[] [15790320, 15790320, 15790320, 15790320, 16777215, 16777215, 15790320, 15790320, 15790320] -> [_ _ _ _ w325]
          tunnel: w279 -> [_ _ _ _ w313]
          tunnel: w276 -> [_ w286 _ _ _]
          frame "Custom", Default {
          }
          frame "Basic" {
            n162 = call <vilib>:"WPI_DashboardUpdateNames.vi"("Controls on Tab"=w286) -> ()  [unwired: 11 in]
          }
          frame "Test" {
            w298 = -2 ("Active Item:Row Number")
            n163 = Index Array(array=w292, index=w291) -> (element=w293:T34)
            n164 = Unbundle(w293) -> ("Operation"=w294:enum16{"Update", "Clear"}, "Color Box"=w295:u32)
            n165 = call <vilib>:"NT Read and Format Entries as Tree.vi"("Operation"=w294, "Name Pattern"=w299, "Tree Refnum"=w300) -> ()  [unwired: 7 in, 2 out]
            n166 = call <vilib>:"NT Read String.vi"("Name"="TestMode/TestName") -> ("String"=w289:string)  [unwired: 9 in, 1 out]
            n167 = case shown="\"\"" w289 {
              tunnel: "TestMode/TestProgress" ("Name") -> [w302 _]
              tunnel: "TestMode/TestProgressText" ("Name") -> [w301 _]
              frame Default {
                n168 = call <vilib>:"NT Read Number.vi"("Name"=w302) -> ("Numeric"=w303:dbl)  [unwired: 9 in, 1 out]
                n169 = call <vilib>:"NT Read String.vi"("Name"=w301) -> ("String"=w304:string)  [unwired: 9 in, 1 out]
                n170 = Bundle("Numeric"=w303, "String"=w304) -> (→"Progress":cluster{"Numeric":dbl, "String":string})  [unwired: 1 in]
              }
              frame "" {
                n171 = local write "Test Name"(u16 0) -> ()
                n172 = property on="Progress" class="Clust (strict)"("Visible"=FALSE) -> ()  [unwired: 2 in, 2 out]
              }
            }
            n173 = property on="Test Tree" class="Tree (strict)"("Active Item Row Number"=w298, "ActiveColNum"=w298, "CellBG"=w295, "Active Item Row Number"=-1 ("Active Item:Row Number"), "CellBG"=u32 5789784 ("Color Box")) -> ()  [unwired: 2 in, 2 out]
          }
          frame "Variables" {
            w310 = string[] ["CameraPublisher", "Usage", "DB"]  # Items to initially close
            n174 = First Call?() -> (First Call?: T/F=w311:bool)
            n175 = control-ref of="Tree"() -> (w312:refnum<vi>)
            n176 = Select(t=w310, s=w311, f=string[] []) -> (s? t:f=w308:string[])
            n177 = call <vilib>:"NT Read and Format Entries as Tree.vi"("Tags to  Close"=w308, "Tree Refnum"=w312) -> ()  [unwired: 8 in, 2 out]
          }
          frame "Commands" {
            w321 = u32 5789784 ("Color Box")
            w322 = T35 {"Row"=-1, "Column"=-2} ("Active Cell:Active Cell")
            w324 = T35 {"Row"=-2, "Column"=-2} ("Active Cell:Active Cell")
            n178 = Index Array(array=w320, index=w319) -> (element=w318:T34)
            n179 = Index Array(array=w325, index=w319) -> (element=w323:u32)
            n180 = local read "Command Selection"() -> (w316:i32)
            n181 = property on="Command Selection" class="MCListbox (strict)"("ActiveCell"=w324, "CellBG"=w323, "ActiveCell"=w322, "CellBG"=w321) -> ()  [unwired: 2 in, 2 out]
            n182 = property on="Command Params" class="Tbl (strict)"("Active Cell"=w324, "Cell BG Color"=w323, "Active Cell"=w322, "Cell BG Color"=w321) -> ()  [unwired: 2 in, 2 out]
            n183 = Unbundle(w318) -> ("Operation"=w317:enum16{"Update", "Clear"})  [unwired: 1 out]
            n184 = call <vilib>:"WPI_DashboardUpdate RPC Info.vi"("Operation"=w317) -> ("update"=w315:bool, "commands"=w314:string[][])  [unwired: 9 in]
            n185 = call <vilib>:"WPI_DashboardUpdate Command Params.vi"("Update"=w315, "NewVal"=w316, "Commands"=w314, "Param Tbl"=w313) -> ()  [unwired: 7 in, 1 out]
            n186 = property on="Command Selection" class="MCListbox (strict)"("ItemNames"=w314) -> ()  [unwired: 2 in, 2 out]
          }
        }
      }
      event "Test Tree": Value Change {
        # "Show appropriate\ncontrols"
        n187 = event-data() -> ("CtlRef"=w330:refnum<vi>, "NewVal"=w328:string)  [unwired: 1 in]
        n188 = property on="Progress" class="Clust (strict)"("Visible"=FALSE) -> ()  [unwired: 2 in, 2 out]
        n189 = call <vilib>:"WPI_UtilitiesGetTreeIOName.vi"("NewVal"=w328, "TreeControl in"=w330) -> ("I/O Name"=w331:string)  [unwired: 9 in]
        n190 = case shown="\"Camera\"" w331 {
          selector: w331 -> [_ w338 _ w360 w369 _]
          tunnel: w328 -> [_ _ w357 w359 _ w376]
          tunnel: cluster{string[]}[] [{["640x480", "320x240", "160x120"]}, {["Auto", "Fixed indoor", "Fixed outdoor 1", "Fixed outdoor 2", "Fixed fluorescent 1", "Fixed fluorescent 2", "Hold current"]}, {["Auto", "Flicker-free 50 Hz", "Flicker-free 60 Hz", "Hold current"]}, {["None", "Prioritize frame rate", "Prioritize image quality"]}, {["Monochrome", "Color"]}] -> [_ _ _ _ _ w375]
          frame Default {
            w333 = FALSE ("Visible")
            w332 = FALSE ("Visible")
            n191 = property on="Test Slider" class="Slide (strict)"("Visible"=w333) -> ()  [unwired: 2 in, 2 out]
            n192 = property on="On/Off" class="Bool (strict)"("Visible"=w333) -> ()  [unwired: 2 in, 2 out]
            n193 = property on="Rev/Fwd" class="Clust (strict)"("Visible"=w333) -> ()  [unwired: 2 in, 2 out]
            n194 = property on="Test Ring" class="Ring (strict)"("Visible"=w332) -> ()  [unwired: 2 in, 2 out]
            n195 = property on="Motor" class="Clust (strict)"("Visible"=w332) -> ()  [unwired: 2 in, 2 out]
          }
          frame "Analog Out", "Motor", "PWM" {
            w339 = FALSE ("Visible")
            n196 = case shown="\"Analog Out\"" w338 {
              tunnel: [1.0 ("Value") -1.0 ("Value") 0.0 ("Value")] -> w337
              tunnel: [255.0 ("Value") 1.0 ("Value") 5.0 ("Value")] -> w336
              tunnel: [128.0 ("Value") 0.0 ("Value") 0.0 ("Value")] -> w335
              tunnel: [64.0 ("Value") 0.5 ("Value") 1.0 ("Value")] -> w334
              frame "PWM" {
              }
              frame "Motor", Default {
              }
              frame "Analog Out" {
              }
            }
            n197 = property on="Test Slider" class="Slide (strict)"("Visible"=w339) -> ()  [unwired: 2 in, 2 out]
            n198 = property on="Test Ring" class="Ring (strict)"("Visible"=w339) -> ()  [unwired: 2 in, 2 out]
            n199 = property on="On/Off" class="Bool (strict)"("Visible"=w339) -> ()  [unwired: 2 in, 2 out]
            n200 = property on="Rev/Fwd" class="Clust (strict)"("Visible"=w339) -> ()  [unwired: 2 in, 2 out]
            n201 = property on="Motor" class="Clust (strict)"("Visible"=TRUE) -> ()  [unwired: 2 in, 2 out]
            n202 = property on="Value" class="Slide (strict)"("Value"=w335, "Scale.Minimum"=w337, "Scale.Maximum"=w336, "Scale.Increment"=w334) -> ()  [unwired: 2 in, 2 out]
          }
          frame "Servo" {
            w355 = FALSE ("Visible")
            n203 = call <vilib>:"NT Read Number.vi"("Name"=w357) -> ("Numeric"=w356:dbl)  [unwired: 9 in, 1 out]
            n204 = property on="Motor" class="Clust (strict)"("Visible"=w355) -> ()  [unwired: 2 in, 2 out]
            n205 = property on="Test Ring" class="Ring (strict)"("Visible"=w355) -> ()  [unwired: 2 in, 2 out]
            n206 = property on="On/Off" class="Bool (strict)"("Visible"=w355) -> ()  [unwired: 2 in, 2 out]
            n207 = property on="Rev/Fwd" class="Clust (strict)"("Visible"=w355) -> ()  [unwired: 2 in, 2 out]
            n208 = property on="Test Slider" class="Slide (strict)"("Visible"=TRUE, "Scale.Maximum"=170.0 ("Scale.Range:Maximum")) -> ()  [unwired: 2 in, 2 out]
            n209 = local write "Test Slider"(w356) -> ()
          }
          frame "Relay", "Solenoid" {
            w358 = FALSE ("Visible")
            n210 = property on="Motor" class="Clust (strict)"("Visible"=w358) -> ()  [unwired: 2 in, 2 out]
            n211 = property on="Test Slider" class="Slide (strict)"("Visible"=w358) -> ()  [unwired: 2 in, 2 out]
            n212 = property on="Test Ring" class="Ring (strict)"("Visible"=w358) -> ()  [unwired: 2 in, 2 out]
            n213 = Search and Replace String(input string=w359, search string="/Value  **", replace string="/Direction") -> (result string=w365:string)  [unwired: 5 in, 3 out]
            n214 = call <vilib>:"NT Read String.vi"("Name"=w365) -> ("String"=w363:string)  [unwired: 9 in, 1 out]
            n215 = Equal?(x="Both directions", y=w363) -> (x = y?=w361:bool)
            n216 = property on="Rev/Fwd" class="Clust (strict)"("Visible"=w361) -> ()  [unwired: 2 in, 2 out]
            n217 = Not(x=w361) -> (.not. x?=w362:bool)
            n218 = property on="On/Off" class="Bool (strict)"("Visible"=w362, "Caption.Text"=w360) -> ()  [unwired: 2 in, 2 out]
          }
          frame "Compressor", "Digital Out" {
            w368 = FALSE ("Visible")
            # "Get direction and finish"
            n219 = property on="Test Ring" class="Ring (strict)"("Visible"=w368) -> ()  [unwired: 2 in, 2 out]
            n220 = property on="Motor" class="Clust (strict)"("Visible"=w368) -> ()  [unwired: 2 in, 2 out]
            n221 = property on="Test Slider" class="Slide (strict)"("Visible"=w368) -> ()  [unwired: 2 in, 2 out]
            n222 = property on="Rev/Fwd" class="Clust (strict)"("Visible"=FALSE) -> ()  [unwired: 2 in, 2 out]
            n223 = property on="On/Off" class="Bool (strict)"("Visible"=TRUE, "Caption.Text"=w369) -> ()  [unwired: 2 in, 2 out]
          }
          frame "Camera" {
            n224 = call <vilib>:"Get Last Path Segment.vi"("String in"=w376) -> ("String out"=w377:string)  [unwired: 10 in]
            n225 = property on="Motor" class="Clust (strict)"("Visible"=FALSE) -> ()  [unwired: 2 in, 2 out]
            n226 = property on="Rev/Fwd" class="Clust (strict)"("Visible"=FALSE) -> ()  [unwired: 2 in, 2 out]
            n227 = case shown="\"White Balance  **\"" w377 {
              tunnel: w376 -> [w383 w392 w401 w410 w419 _ w425]
              tunnel: w375 -> [w381 w389 w398 w407 w416 _ _]
              frame "Size  **" {
                n228 = Index Array(array=w381) -> (element=w380:cluster{string[]})  [unwired: 1 in]
                n229 = call <vilib>:"NT Read String.vi"("Name"=w383) -> ("String"=w382:string)  [unwired: 9 in, 1 out]
                n230 = property on="Test Slider" class="Slide (strict)"("Visible"=FALSE) -> ()  [unwired: 2 in, 2 out]
                n231 = property on="Test Ring" class="Ring (strict)"("Visible"=TRUE) -> ()  [unwired: 2 in, 2 out]
                n232 = Unbundle(w380) -> (w378:string[])
                n233 = Match First String(2:w378, 3:w382) -> (0:w379:i32)  [unwired: 1 out]
                n234 = property on="Test Ring" class="Ring (strict)"("Value"=w379, "Strings []"=w378) -> ()  [unwired: 2 in, 2 out]
              }
              frame "White Balance  **" {
                n235 = call <vilib>:"NT Read String.vi"("Name"=w392) -> ("String"=w391:string)  [unwired: 9 in, 1 out]
                n236 = Index Array(array=w389, index=1) -> (element=w390:cluster{string[]})
                n237 = property on="Test Slider" class="Slide (strict)"("Visible"=FALSE) -> ()  [unwired: 2 in, 2 out]
                n238 = property on="Test Ring" class="Ring (strict)"("Visible"=TRUE) -> ()  [unwired: 2 in, 2 out]
                n239 = Unbundle(w390) -> (w387:string[])
                n240 = Match First String(2:w387, 3:w391) -> (0:w386:i32)  [unwired: 1 out]
                n241 = property on="Test Ring" class="Ring (strict)"("Value"=w386, "Strings []"=w387) -> ()  [unwired: 2 in, 2 out]
              }
              frame "Exposure  **" {
                n242 = call <vilib>:"NT Read String.vi"("Name"=w401) -> ("String"=w400:string)  [unwired: 9 in, 1 out]
                n243 = Index Array(array=w398, index=2) -> (element=w399:cluster{string[]})
                n244 = property on="Test Slider" class="Slide (strict)"("Visible"=FALSE) -> ()  [unwired: 2 in, 2 out]
                n245 = property on="Test Ring" class="Ring (strict)"("Visible"=TRUE) -> ()  [unwired: 2 in, 2 out]
                n246 = Unbundle(w399) -> (w395:string[])
                n247 = Match First String(2:w395, 3:w400) -> (0:w396:i32)  [unwired: 1 out]
                n248 = property on="Test Ring" class="Ring (strict)"("Value"=w396, "Strings []"=w395) -> ()  [unwired: 2 in, 2 out]
              }
              frame "Exposure Priority  **" {
                n249 = call <vilib>:"NT Read String.vi"("Name"=w410) -> ("String"=w409:string)  [unwired: 9 in, 1 out]
                n250 = Index Array(array=w407, index=3) -> (element=w408:cluster{string[]})
                n251 = property on="Test Slider" class="Slide (strict)"("Visible"=FALSE) -> ()  [unwired: 2 in, 2 out]
                n252 = property on="Test Ring" class="Ring (strict)"("Visible"=TRUE) -> ()  [unwired: 2 in, 2 out]
                n253 = Unbundle(w408) -> (w404:string[])
                n254 = Match First String(2:w404, 3:w409) -> (0:w405:i32)  [unwired: 1 out]
                n255 = property on="Test Ring" class="Ring (strict)"("Value"=w405, "Strings []"=w404) -> ()  [unwired: 2 in, 2 out]
              }
              frame "Color Enable  **" {
                n256 = call <vilib>:"NT Read String.vi"("Name"=w419) -> ("String"=w418:string)  [unwired: 9 in, 1 out]
                n257 = Index Array(array=w416, index=4) -> (element=w417:cluster{string[]})
                n258 = property on="Test Slider" class="Slide (strict)"("Visible"=FALSE) -> ()  [unwired: 2 in, 2 out]
                n259 = property on="Test Ring" class="Ring (strict)"("Visible"=TRUE) -> ()  [unwired: 2 in, 2 out]
                n260 = Unbundle(w417) -> (w413:string[])
                n261 = Match First String(2:w413, 3:w418) -> (0:w414:i32)  [unwired: 1 out]
                n262 = property on="Test Ring" class="Ring (strict)"("Value"=w414, "Strings []"=w413) -> ()  [unwired: 2 in, 2 out]
              }
              frame Default {
                n263 = property on="Test Slider" class="Slide (strict)"("Visible"=FALSE) -> ()  [unwired: 2 in, 2 out]
                n264 = property on="Test Ring" class="Ring (strict)"("Visible"=FALSE) -> ()  [unwired: 2 in, 2 out]
              }
              frame "Brightness  **", "Color Level  **", "Compression  **", "FPS  **", "Sharpness  **" {
                n265 = call <vilib>:"NT Read Number.vi"("Name"=w425) -> ("Numeric"=w424:dbl)  [unwired: 9 in, 1 out]
                n266 = property on="Test Ring" class="Ring (strict)"("Visible"=FALSE) -> ()  [unwired: 2 in, 2 out]
                n267 = property on="Test Slider" class="Slide (strict)"("Visible"=TRUE, "Scale.Maximum"=100.0 ("Scale.Range:Maximum")) -> ()  [unwired: 2 in, 2 out]
                n268 = local write "Test Slider"(w424) -> ()
              }
            }
            n269 = property on="On/Off" class="Bool (strict)"("Visible"=FALSE) -> ()  [unwired: 2 in, 2 out]
          }
        }
      }
      event "Test Name": Mouse Enter {
        # "Populate the ring with the list of tests"
        n270 = event-data() -> ()  [unwired: 1 in, 1 out]
        n271 = call <vilib>:"NT Read String Array.vi"("Name"="TestMode/TestList") -> ("String Array"=w433:string[])  [unwired: 9 in, 1 out]
        n272 = Build Array (concatenate)("Select the test to run...", w433) -> (w432:string[])
        n273 = property on="Test Name" class="Ring (strict)"("Strings []"=w432) -> ()  [unwired: 2 in, 2 out]
      }
      event "Test Name": Value Change {
        w435 = FALSE ("Visible")
        # "Tell the robot the test name to run"
        n274 = event-data() -> ("NewVal"=w439:u16)  [unwired: 1 in]
        n275 = property on="Test Name" class="Ring (strict)"() -> ("Strings []"=w440:string[])  [unwired: 2 in, 2 out]
        n276 = property on="Test Ring" class="Ring (strict)"("Visible"=w435) -> ()  [unwired: 2 in, 2 out]
        n277 = property on="Motor" class="Clust (strict)"("Visible"=w435) -> ()  [unwired: 2 in, 2 out]
        n278 = property on="Test Slider" class="Slide (strict)"("Visible"=w435) -> ()  [unwired: 2 in, 2 out]
        n279 = property on="On/Off" class="Bool (strict)"("Visible"=w435) -> ()  [unwired: 2 in, 2 out]
        n280 = property on="Rev/Fwd" class="Clust (strict)"("Visible"=w435) -> ()  [unwired: 2 in, 2 out]
        n281 = property on="Progress" class="Clust (strict)"("Visible"=TRUE) -> ()  [unwired: 2 in, 2 out]
        n282 = local write "Progress"(T9 {"Test Progress"=0, "Test Progress Text"=""} ("Progress")) -> ()
        n283 = Index Array(array=w440, index=w439) -> (element=w438:string)
        n284 = call <vilib>:"NT Write String.vi"("String"=w438, "Name"="TestMode/TestName") -> ()  [unwired: 9 in, 1 out]
      }
      event "Select Auto": Mouse Enter {
        # "Populate the combo box with the list of autonomous options"
        n285 = event-data() -> ()  [unwired: 1 in, 1 out]
        n286 = call <vilib>:"NT Read String Array.vi"("Name"="Auto List") -> ("String Array"=w442:string[])  [unwired: 9 in, 1 out]
        n287 = property on="Select Auto" class="CmbBox"("Strings[]"=w442) -> ()  [unwired: 2 in, 2 out]
      }
      event "Select Auto": Value Change {
        # "User modified the Auto Selection. Write to NT variable so robot knows."
        n288 = event-data() -> ("NewVal"=w445:string)  [unwired: 1 in]
        n289 = call <vilib>:"NT Write String.vi"("String"=w445, "Name"="Auto Selector") -> ()  [unwired: 9 in, 1 out]
      }
      event "Command Selection": Value Change {
        # "Get the params and show in table"
        n290 = event-data() -> ("NewVal"=w451:i32)  [unwired: 1 in]
        n291 = property on="Command Selection" class="MCListbox (strict)"() -> ("ItemNames"=w449:string[][])  [unwired: 2 in, 2 out]
        n292 = call <vilib>:"WPI_DashboardUpdate Command Params.vi"("NewVal"=w451, "Commands"=w449, "Param Tbl"=w450) -> ()  [unwired: 8 in, 1 out]
      }
      event "Execute Command": Value Change {
        # "Started one, Unique ID holds\nresponse"
        n293 = event-data() -> ()  [unwired: 1 in, 1 out]
        n294 = property on="Command Selection" class="MCListbox (strict)"() -> ("ItemNames"=w462:string[][])  [unwired: 2 in, 2 out]
        n295 = Index Array(array=w462, index (row)="Command Selection", index (col)=0) -> (element=w460:string)
        n296 = call <vilib>:"Invoke Commands.vi"("Command Params"="Command Params", "Function Name"=w460) -> ("Params"=w456:u8, "Started"=w455:bool)  [unwired: 7 in, 1 out]
        n297 = Array Subset(array="Command Params", length (row)=w456) -> (w457:string[][])  [unwired: 3 in]
        n298 = Select(t="Executing" ("Cmd Status"), s=w455, f="" ("Cmd Status")) -> (s? t:f=→"Cmd Status":string)
      }
      event "Command Selection": Double Click {
        n299 = event-data() -> ("Row"=w470:i32)  [unwired: 1 in]
        n300 = property on="Command Selection" class="MCListbox (strict)"() -> ("ItemNames"=w473:string[][])  [unwired: 2 in, 2 out]
        n301 = local read "Command Params"() -> (w469:string[][])
        n302 = Index Array(array=w473, index (row)=w470, index (col)=0) -> (element=w471:string)
        n303 = call <vilib>:"Invoke Commands.vi"("Command Params"=w469, "Function Name"=w471) -> ("Params"=w468:u8, "Started"=w463:bool)  [unwired: 7 in, 1 out]
        n304 = Array Subset(array=w469, length (row)=w468) -> (w467:string[][])  [unwired: 3 in]
        n305 = Select(t="Executing" ("Cmd Status"), s=w463, f="" ("Cmd Status")) -> (s? t:f=w464:string)
        n306 = local write "Cmd Status"(w464) -> ()
      }
      event "CheckList": Double Click {
        # "Shift clears all"
        # "Update symbols on the listbox"
        n307 = event-data() -> ("PlatMods.Shift"=w475:bool, "Row"=w477:i32)  [unwired: 1 in]
        n308 = case shown="True" w475 {
          tunnel: w477 -> [w481 _]
          tunnel: 1 -> [w480 _]
          frame False {
            n309 = property on="CheckList" class="LstBox (strict)"() -> ("Item Symbols"=w479:i32[])  [unwired: 2 in, 2 out]
            n310 = Replace Array Subset(array=w479, new element=w480, index=w481) -> (w478:i32[])
            n311 = property on="CheckList" class="LstBox (strict)"("Item Symbols"=w478) -> ()  [unwired: 2 in, 2 out]
          }
          frame True {
            w482 = 0 ("Top Row")
            n312 = property on="CheckList" class="LstBox (strict)"() -> ("Number of Rows"=w484:u32)  [unwired: 2 in, 2 out]
            n313 = Initialize Array(0, w484) -> (w483:i32[])
            n314 = property on="CheckList" class="LstBox (strict)"("Top Row"=w482, "Value"=w482, "Item Symbols"=w483) -> ()  [unwired: 2 in, 2 out]
          }
        }
      }
      event "CheckList": Key Down {
        # "Update symbols on the listbox\nLeft and right keys check and uncheck"
        n315 = event-data() -> ("VKey"=w488:T32)  [unwired: 1 in]
        n316 = case shown="\"Left\", \"Right\"" w488 {
          selector: w488 -> [w493 _]
          tunnel: eventvkey."Left" ("VKey") -> [w491 _]
          frame "Left", "Right" {
            n317 = Equal?(x=w491, y=w493) -> (x = y?=w492:bool)
            n318 = Select(t=0, s=w492, f=1) -> (s? t:f=w494:i32)
            n319 = property on="CheckList" class="LstBox (strict)"() -> ("Item Symbols"=w497:i32[])  [unwired: 2 in, 2 out]
            n320 = Replace Array Subset(array=w497, new element=w494, index="CheckList") -> (w496:i32[])
            n321 = property on="CheckList" class="LstBox (strict)"("Item Symbols"=w496) -> ()  [unwired: 2 in, 2 out]
          }
          frame Default {
          }
        }
      }
      event "Motor.Enable": Value Change {
        # "When the test mode otor enable helper is set, update that\ntree row item's value"
        n322 = event-data() -> ("NewVal"=w503:bool)  [unwired: 1 in]
        n323 = Unbundle("Motor") -> ("Value"=w502:dbl)  [unwired: 1 out]
        n324 = Select(t=w502, s=w503, f=0.0) -> (s? t:f=w500:dbl)
        n325 = call <vilib>:"NT Write Number.vi"("Numeric"=w500, "Name"=w499) -> ()  [unwired: 9 in, 1 out]
      }
      event "Test Slider": Value Change {
        # "When the test mode slider helper is set, update that\ntree row item's value"
        n326 = event-data() -> ("NewVal"=w506:dbl)  [unwired: 1 in]
        n327 = call <vilib>:"NT Write Number.vi"("Numeric"=w506, "Name"=w507) -> ()  [unwired: 9 in, 1 out]
      }
      event "On/Off": Value Change {
        # "When the test mode on/off helper value is set, update that\ntree row item's value"
        n328 = event-data() -> ("NewVal"=w511:bool)  [unwired: 1 in]
        n329 = Boolean To (0,1)(Boolean=w511) -> (0, 1=w510:i16)
        n330 = call <vilib>:"NT Write Number.vi"("Numeric"=w510, "Name"=w509) -> ()  [unwired: 9 in, 1 out]
      }
      event "Rev/Fwd": Value Change {
        # "When the test mode helper value for relays is set, update that\ntree row item's value"
        n331 = event-data() -> ("NewVal.Forward"=w519:bool, "NewVal.Reverse"=w518:bool)  [unwired: 1 in]
        n332 = Boolean To (0,1)(Boolean=w519) -> (0, 1=w515:i16)
        n333 = Boolean To (0,1)(Boolean=w518) -> (0, 1=w517:i16)
        n334 = Negate(x=w517) -> (-x=w516:i16)
        n335 = Add(x=w515, y=w516) -> (x+y=w514:i16)
        n336 = call <vilib>:"NT Write Number.vi"("Numeric"=w514, "Name"=w513) -> ()  [unwired: 9 in, 1 out]
      }
      event "Test Ring": Value Change {
        # "When a test mode helper value is selected from the ring,\nset the tree item's variable to the string value"
        n337 = event-data() -> ("NewVal"=w523:u16)  [unwired: 1 in]
        n338 = property on="Test Ring" class="Ring (strict)"() -> ("Strings []"=w524:string[])  [unwired: 2 in, 2 out]
        n339 = Index Array(array=w524, index=w523) -> (element=w522:string)
        n340 = call <vilib>:"NT Write String.vi"("String"=w522, "Name"=w521) -> ()  [unwired: 9 in, 1 out]
      }
      event "Rec Mode": Value Change {
        # "Update globals for recording mode and path to read log from.\nClear when logging and let NetworkTables set path for vision to\nuse."
        n341 = event-data() -> ("NewVal"=w535:enum32{"Stop", "Record", "Playback"})  [unwired: 1 in]
        n342 = global write "WPI_DashboardLogging Global.vi" "Logging Filename"(path "") -> ()
        n343 = global write "WPI_DashboardLogging Global.vi" "Recording"(w535) -> ()
        n344 = case shown="\"Playback\"" w535 {
          tunnel: w534 -> [_ w537 w546]
          tunnel: [_ _ w545] -> w532
          tunnel: [_ _ w544] -> _
          tunnel: w530 -> [_ _ w542]
          tunnel: cluster{i32, i32} {-250, 170} -> [_ _ w541]
          tunnel: [_ _ T33 {"Image Size"=TRUE, "Image Type"=TRUE, "Pixel Value"=TRUE, "ROI Information"=TRUE, "Zoom Factor"=FALSE} ("Image Information Shown:All Elements")] -> w525
          tunnel: [_ _ TRUE ("Zoom Factor")] -> w526
          tunnel: w528 -> [_ _ w538]
          frame Default {
          }
          frame "Stop", "Record" {
            # "Place Window too"
            n345 = invoke class="VI" method="FP.Close"(reference=w537) -> (reference out=w536:refnum<vi>)  [unwired: 2 in, 2 out]
            n346 = invoke class="VI" method="Abort VI"(reference=w536) -> ()  [unwired: 2 in, 3 out]
          }
          frame "Playback" {
            n347 = call "Open Playback Panel.vi"("Offset"=w541, "DB VI Ref"=w542, "Playback in"=w546) -> ("Playback out"=w543:refnum<vi>)  [unwired: 8 in]
            n348 = register-events(w543, w538) -> (reference out=w545:refnum<event-registration>, error out=w544:errorcluster)  [unwired: 2 in]
          }
        }
        n349 = call <vilib>:"WPI_DashboardNT Log FieldName Cache.vi"("Operation"=enum16{"Lookup/Add", "Index", "Clear"}."Clear") -> ()  [unwired: 8 in, 3 out]
        n350 = property on="Camera Image" class="ImageControl"("Image Information Shown"=w525, "Image Information Visible"=w526) -> ()  [unwired: 2 in, 2 out]
        n351 = property on="Camera Image Right" class="ImageControl"("Image Information Shown"=w525, "Image Information Visible"=w526) -> ()  [unwired: 2 in, 2 out]
      }
      event Panel Close {
        w548 = enum32{"Stop", "Record", "Playback"}."Stop" ("Rec Mode")
        # "Playback window has been closed, abort"
        n352 = event-data() -> ()  [unwired: 1 in, 4 out]
        n353 = local write "Rec Mode"(w548) -> ()
        n354 = global write "WPI_DashboardLogging Global.vi" "Recording"(w548) -> ()
      }
      event Panel Close {
        # "Abort playback window and ourself"
        n355 = event-data() -> ()  [unwired: 1 in, 4 out]
        n356 = invoke class="VI" method="FP.Close"(reference=w552) -> (reference out=w551:refnum<vi>)  [unwired: 2 in, 2 out]
        n357 = invoke class="VI" method="Abort VI"(reference=w551) -> (error out=w550:errorcluster)  [unwired: 2 in, 2 out]
        n358 = invoke class="VI" method="Abort VI"(error in=w550) -> ()  [unwired: 2 in, 3 out]
      }
      event User Event {
        n359 = event-data() -> ("IDs"=w559:cluster{"RPC field ID":u16, "Unique ID":u16}, "String"=w558:string)  [unwired: 1 in]
        n360 = local write "Cmd Status"("" ("Cmd Status")) -> ()
        n361 = Bundle("IDs"=w559, "String"=w558) -> (w557:T12)  [unwired: 1 in]
        n362 = call <vilib>:"Retrieve RPC Response.vi"("RPC Response"=w557) -> ("Output"=w555:string[][])  [unwired: 10 in]
        n363 = Build Array (concatenate)(w553, w555) -> (w554:string[][])
        n364 = local write "Command Params"(w554) -> ()
      }
      event "Tree": Double Click {
        n365 = event-data() -> ("PlatMods"=w565:T36, "Tag"=w562:string)  [unwired: 1 in]
        n366 = Unbundle(w565) -> ("Shift"=w564:bool)  [unwired: 4 out]
        n367 = Not(x=w564) -> (.not. x?=w563:bool)
        n368 = String Subset(string=w562, length (rest)=1 ("length (rest)")) -> (substring=w561:string)  [unwired: 1 in]
        n369 = case shown="\"/\"" w561 {
          tunnel: w562 -> [_ w568]
          tunnel: w563 -> [_ w567]
          frame Default {
          }
          frame "/" {
            n370 = call <vilib>:"NT Update Persistence.vi"("Persistence"=w567, "Name"=w568) -> ()  [unwired: 9 in, 1 out]
          }
        }
      }
    }
  }
  n371 = while {
    tunnel: w56 -> [w580]
    tunnel: w1 -> [w578]
    tunnel: [w576] -> _
    tunnel: u32 1000 ("milliseconds to wait") -> [w575]
    tunnel: w27 -> [w569]
    i -> [w576]
    stop <- FALSE stop-if-true
    n372 = Wait on Notification(notifier=w578, timeout in ms (-1)=w575) -> (notification=w577:string, timed out?=w573:bool)  [unwired: 2 in, 2 out]
    n373 = local read "Rec Mode"() -> (w571:enum32{"Stop", "Record", "Playback"})
    n374 = Equal?(x=w571, y=u16 2 ("Rec Mode")) -> (x = y?=w572:bool)
    n375 = Compound Arithmetic op=OR(invert w573, w572) -> (w574:bool)
    n376 = case shown="True" w574 {
      tunnel: w580 -> [_ w583]
      tunnel: w577 -> [_ w582]
      tunnel: w569 -> [_ w581]
      frame False {
      }
      frame True {
        n377 = call <vilib>:"Bind Controls to SmartDashboard.vi"("RPC ref"=w581, "Bound Control Refs"=w583, "Server IP Address"=w582) -> ()  [unwired: 9 in]
      }
    }
  }
